vi "show contracts.vi"(8 "error in":errorcluster, 11 "Data Cluster in":T1) -> (0 "error out":errorcluster, 2 "Response body":string, 3 "Data Cluster out":T1)   [LabVIEW 2024, in "GUI.lvlib" / "Functions.lvlib"]
uses:
  Functions.lvlib
  Module Data--cluster.ctl
  <vilib>/addons/_JKI.lib/REST Client/classes/REST Client/REST Client.lvclass
  GUI.lvlib
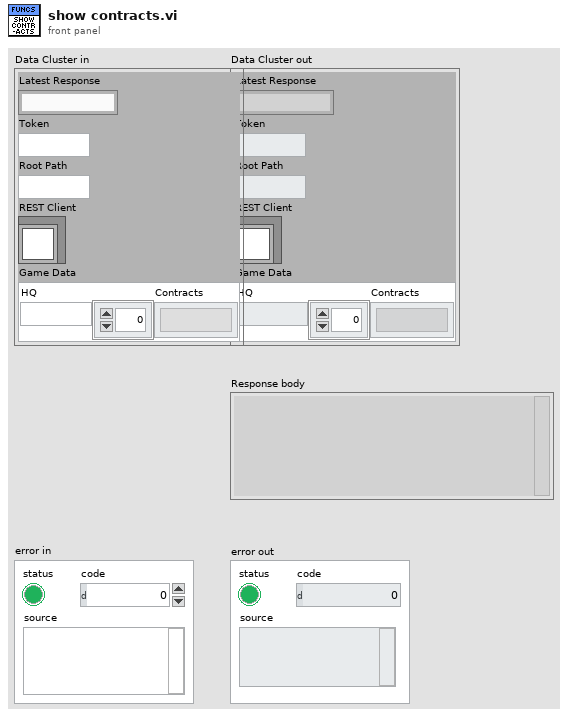
[diagram p1: front panel]
types:
  T1 = typedef "GUI.lvlib/Module Data--cluster.ctl" = cluster{"Latest Response":string, "Token":string, "Root Path":string, "REST Client":refnum<class "REST Client.lvclass">, "Game Data":cluster{"HQ":string, "Contracts":string[]}}
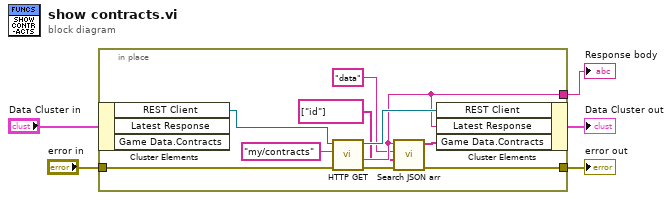
[diagram p0: block diagram]
diagram:
  n1 = in-place {
    in-place-border: [w6] -> w2
    in-place-border: [w11] -> w3
    in-place-border: "error in" -> [w12]
    n2 = in-place-cluster #1("Data Cluster in") -> ("REST Client"=w14:refnum<class "REST Client.lvclass">)  [unwired: 2 out]
    n3 = call-dynamic "HTTP GET.vi"("error in (no error)"=w12, "Path"="my/contracts", "REST Client in"=w14) -> ("error out"=w7:errorcluster, "Response body"=w11:string, "REST Client out"=w13:refnum<class "REST Client.lvclass">)  [unwired: 3 in, 3 out]
    n4 = call "Search JSON arr.vi"("error in"=w7, "Search Terms"=string[] ["id"], "Name of arr"="data", "Response body"=w11) -> ("error out"=w6:errorcluster, "Respsonse"=w8:string[])  [unwired: 6 in]
    n5 = in-place-cluster #1("REST Client"=w13, "Latest Response"=w11, "Game Data.Contracts"=w8) -> (→"Data Cluster out":T1)
  }
  "error out" <- w2
  "Response body" <- w3
